vi "Status Current Status.vi"(5 "Retry Attempts (0)":i32 min=0, 7 "Fast Comms (F)":bool, 8 "error in (no error)":errorcluster, 11 "VISA resource name":refnum<visa-resource-name>) -> (0 "error out":errorcluster, 2 "Status Cluster":T1, 3 "VISA resource name out":refnum<visa-resource-name>)   [LabVIEW 2020, in "ChromTech Series I Drivers.lvlib"]
doc: "Returns the flow rate in ml/min, upper pressure limit, lower pressure limit, pressure units, and the run/stop state, where True = running and False = stopped.\n\nFor Series I, the upper and lower pressure limits are always zero."
uses:
  <instrlib>/RxnRover/ChromtechSeriesIDriver/ChromTech Series I Drivers.lvlib
panel:
  out "Response":string
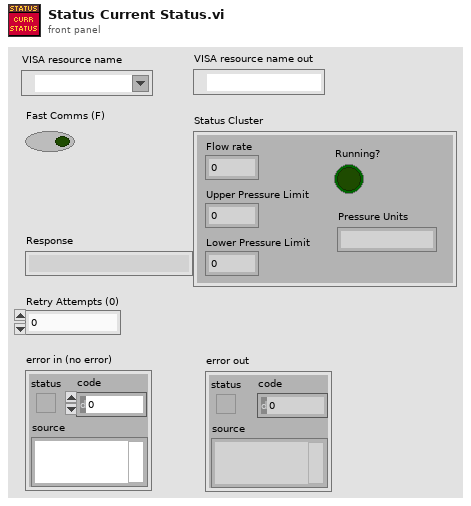
[diagram p1: front panel]
types:
  T1 = cluster{"Flow rate":dbl, "Upper Pressure Limit":dbl, "Lower Pressure Limit":dbl, "Pressure Units":string, "Running?":bool}
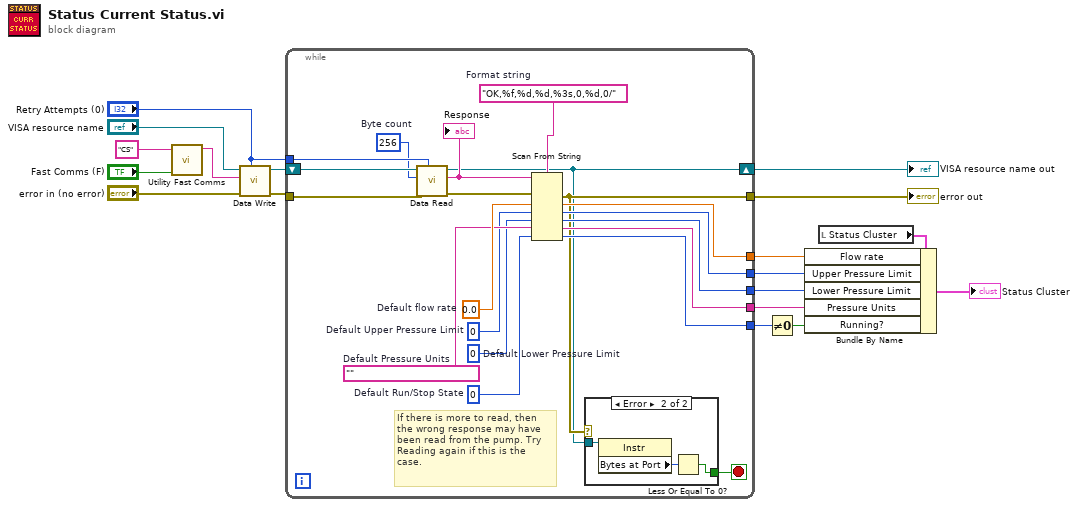
[diagram p0: block diagram]
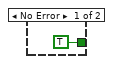
[diagram p2: hidden frame]
diagram:
  n1 = call <instrlib>:"Utility Fast Comms.vi"("Fast Comms"="Fast Comms (F)", "Command"="CS" ("command")) -> ("Fast Command"=w13:string)  [unwired: 9 in]
  n2 = call <instrlib>:"Data Write.vi"("Retry Attempts (0)"="Retry Attempts (0)", "error in (no error)"="error in (no error)", "Command"=w13, "VISA Refnum in"="VISA resource name") -> ("error out"=w4:errorcluster, "VISA Refnum out"=w3:refnum<visa-resource-name>)  [unwired: 6 in]
  n3 = while {
    tunnel: [w38] -> w14
    tunnel: [w37] -> w10
    tunnel: [w36] -> w9
    tunnel: [w35] -> w8
    tunnel: [w34] -> w7
    tunnel: "Retry Attempts (0)" -> [w33]
    shift-right: [w20] -> w1
    shift-left: w3 -> [w31]
    tunnel: w4 -> [w32]
    tunnel: [w21] -> w2
    stop <- w19 stop-if-true
    w22 = u32 256  # Byte count
    w24 = 0  # Default Lower Pressure Limit
    w25 = 0  # Default Upper Pressure Limit
    w26 = 0  # Default Run/Stop State
    w27 = ""  # Default Pressure Units
    w28 = 0.0  # Default flow rate
    w30 = "OK,%f,%d,%d,%3s,0,%d,0/"  # Format string
    # "If there is more to read, then\nthe wrong response may have\nbeen read from the pump. Try\nReading again if this is the\ncase."
    n4 = call <instrlib>:"Data Read.vi"("Retry Attempts (0)"=w33, "error in (no error)"=w32, "Bytes to read"=w22, "VISA Refnum in"=w31) -> ("error out"=w29:errorcluster, "read buffer"=w23:string, "VISA Refnum out"=w20:refnum<visa-resource-name>)  [unwired: 5 in]
    "Response" <- w23
    n5 = Scan From String(format string=w30, input string=w23, error in=w29, default 1=w28, default 2=w25, default 3=w24, default 4=w27, default 5=w26) -> (error out=w21:errorcluster, output 1=w34:dbl, output 2=w35:i32, output 3=w36:i32, output 4=w37:string, output 5=w38:i32)  [unwired: 1 in, 2 out]
    n6 = case shown="Error" w21 {
      tunnel: w20 -> [_ w42]
      tunnel: [TRUE w40] -> w19
      frame No Error {
      }
      frame Error {
        n7 = property class="Instr"(reference=w42) -> ("Bytes at Port"=w41:u32)  [unwired: 1 in, 2 out]
        n8 = Less Or Equal To 0?(x=w41) -> (x <= 0?=w40:bool)
      }
    }
  }
  "VISA resource name out" <- w1
  "error out" <- w2
  n9 = Not Equal To 0?(x=w14) -> (x != 0?=w11:bool)
  n10 = local read "Status Cluster"() -> (w12:T1)
  n11 = Bundle By Name(cluster=w12, "Flow rate"=w7, "Upper Pressure Limit"=w8, "Lower Pressure Limit"=w9, "Pressure Units"=w10, "Running?"=w11) -> (→"Status Cluster":T1)
